vi "Default Path.vi"(8 "error in (no error)":errorcluster, 11 "PuTTY Client in":refnum<class "PuTTY Client.lvclass">) -> (0 "error out":errorcluster, 2 "path":path, 3 "PuTTY Client out":refnum<class "PuTTY Client.lvclass">)   [LabVIEW 2020, in "NI_SSH.lvlib" / "PuTTY Client.lvclass"]
uses:
  <vilib>/net/SSH/Client/PuTTY/PuTTY Client.lvclass
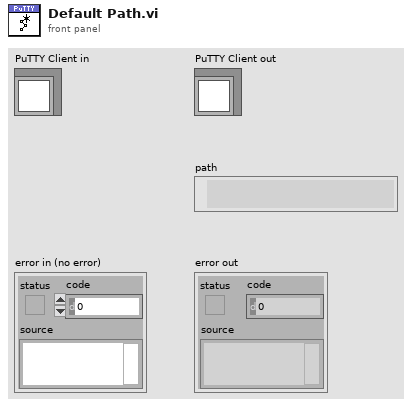
[diagram p1: front panel]
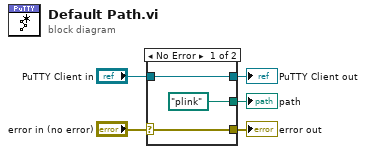
[diagram p0: block diagram]
diagram:
  n1 = case shown="No Error" "error in (no error)" {
    selector: "error in (no error)" -> [w7 w10]
    tunnel: [w7 w10] -> w2
    tunnel: [w8 w9] -> w3
    tunnel: "PuTTY Client in" -> [w8 w9]
    tunnel: [path "plink" ("path") _] -> w1
    frame No Error {
    }
    frame Error {
    }
  }
  "error out" <- w2
  "PuTTY Client out" <- w3
  "path" <- w1
